vi "FPGA.vi"() -> ()   [LabVIEW 2020]
uses:
  <vilib>/rvi/eio/common/nirviEmuTemplateMethod_errors.vi
  <vilib>/rvi/Emulation/niFpgaGetClockAttributes.vi
  <vilib>/rvi/Emulation/niFpgaSctlEmulationGetInTimedLoop.vi
  <vilib>/rvi/Emulation/niFpgaEmulationReportErrorSimple.vi
  <vilib>/rvi/interface/RandomDataEmulation/niFpgaRandomDataHandleErrors.vi
  <vilib>/rvi/Emulation/niFpgaCriticalErrorInLSC.vi
  <vilib>/eio/EIONode/EIONode.xnode
  <vilib>/rvi/DataTransferAndStorage/Container/XNode/niFpgaContainer.xnode
  <vilib>/rvi/interface/RandomDataEmulation/nirviRandomDataFpgaReadWriteTemplate.vi
panel:
  out "single precision float":sgl
  out "appended array":fxp<+/-,24,7>[](array[numeric])
  out "Actual loop rate":u32
  in  "Rate (uSec)":u32 caption="Count(uSec)"
  out "Timed Out?":bool
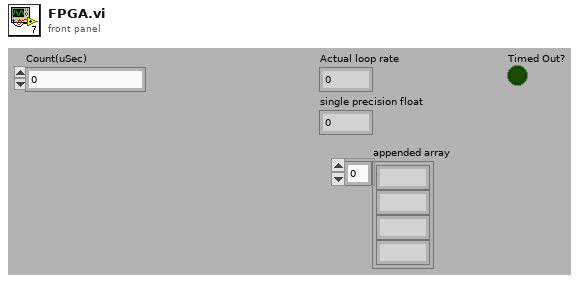
[diagram p1: front panel]
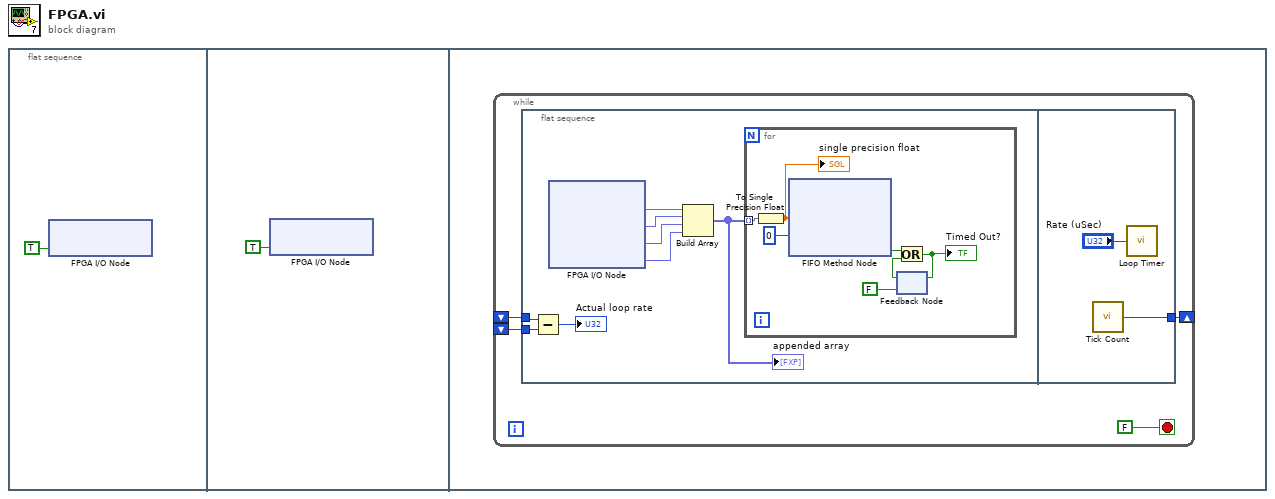
[diagram p0: block diagram]
diagram:
  n1 = flat-sequence {
    frame #0 {
      n2 = xnode "FPGA I/O Node"("Mod1/Stop"=TRUE) -> ()  [unwired: 1 in, 1 out]
    }
    frame #1 {
      n3 = xnode "FPGA I/O Node"("Mod1/Start"=TRUE) -> ()  [unwired: 1 in, 1 out]
    }
    frame #2 {
      n4 = while {
        shift-right: [w5] -> _
        shift-left: _ -> [w4]
        shift-left: _ -> [w3]
        stop <- FALSE stop-if-true
        n5 = flat-sequence {
          tunnel: w4 -> [w9]
          tunnel: w3 -> [w8]
          tunnel: [w22] -> w5
          frame #0 {
            n6 = Subtract(x=w9, y=w8) -> (x-y=→"Actual loop rate":u32)
            n7 = xnode "FPGA I/O Node"() -> ("Mod1/AI0"=w14:fxp<+/-,24,7>, "Mod1/AI1"=w13:fxp<+/-,24,7>, "Mod1/AI2"=w12:fxp<+/-,24,7>, "Mod1/AI3"=w11:fxp<+/-,24,7>)  [unwired: 4 in, 4 out]
            n8 = Build Array(w14, w13, w12, w11) -> (w10:fxp<+/-,24,7>[])
            "appended array" <- w10
            n9 = for {
              tunnel: w10 -> [w16] mode=indexing
              n10 = To Single Precision Float(number=w16) -> (single precision float=w15:sgl)
              "single precision float" <- w15
              n11 = xnode ("FIFO Method Node")("Element"=w15, "Timeout"=0) -> ("Timed Out?"=w20:bool)  [unwired: 1 in, 1 out]
              n12 = feedback #1(FALSE) -> (w19:bool)
              n13 = Or(x=w20, y=w19) -> (x .or. y?=w18:bool)
              "Timed Out?" <- w18
              n14 = feedback-in #1(w18) -> ()
            }
          }
          frame #1 {
            n15 = call "Tick Count"() -> ("Tick Count(uSec)"=w22:u32)
            n16 = call "Loop Timer"("Count(uSec)"="Rate (uSec)") -> ()  [unwired: 1 out]
          }
        }
      }
    }
  }
